vi "Thorlabs-Time Out Check.vi"(8 "error in (no error)":errorcluster, 11 "pDataBuffer in":u16[](array[numeric])) -> (0 "error out":errorcluster, 3 "pDataBuffer out":u16[](array[numeric]))   [LabVIEW 2020]
uses:
  LSM_SDK/ThorConfocal.lvlib
  ECU_SDK/ThorECU.lvlib
panel:
  # "Check that the connection to the scanner is OK"
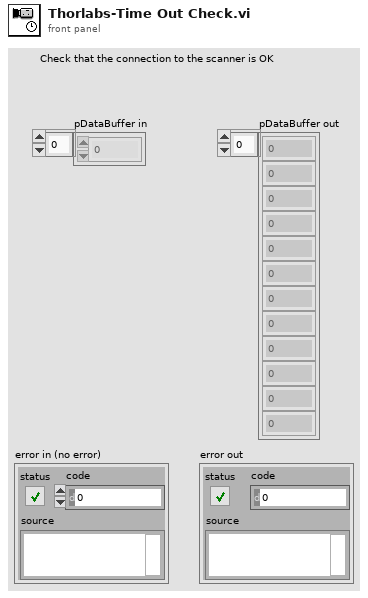
[diagram p1: front panel]
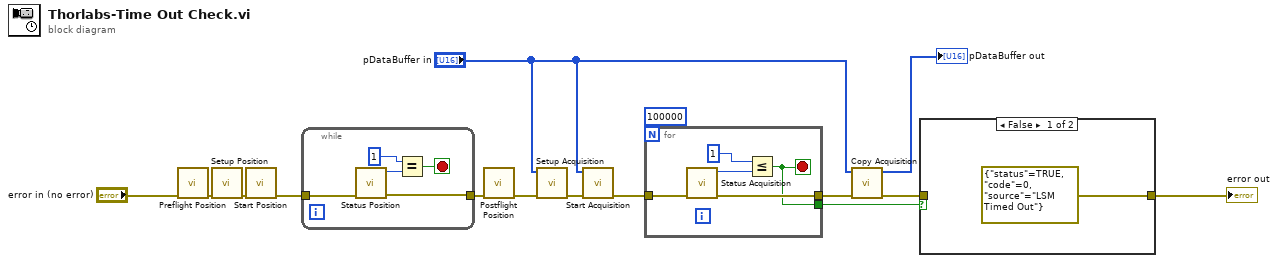
[diagram p0: block diagram]
diagram:
  n1 = call "Preflight Position.vi"("error in (no error)"="error in (no error)") -> ("error out"=w10:errorcluster)  [unwired: 9 in, 1 out]
  n2 = call "Setup Position.vi"("error in (no error)"=w10) -> ("error out"=w11:errorcluster)  [unwired: 9 in, 1 out]
  n3 = call "Start Position.vi"("error in (no error)"=w11) -> ("error out"=w9:errorcluster)  [unwired: 9 in, 1 out]
  n4 = while {
    tunnel: w9 -> [w20]
    tunnel: [w19] -> w8
    stop <- w17 stop-if-true
    n5 = call "Status Position.vi"("error in (no error)"=w20) -> ("error out"=w19:errorcluster, "status out"=w16:i32)  [unwired: 8 in, 1 out]
    n6 = Equal?(x=1, y=w16) -> (x = y?=w17:bool)
  }
  n7 = call "Postflight Position.vi"("error in (no error)"=w8) -> ("error out"=w7:errorcluster)  [unwired: 9 in, 1 out]
  n8 = call "Setup Acquisition.vi"("error in (no error)"=w7, "pDataBuffer"="pDataBuffer in") -> ("error out"=w13:errorcluster)  [unwired: 3 in, 2 out]
  n9 = call "Start Acquisition.vi"("error in (no error)"=w13, "pDataBuffer"="pDataBuffer in") -> ("error out"=w12:errorcluster)  [unwired: 3 in, 2 out]
  n10 = for {
    N: 100000 ("x") -> [_]
    tunnel: [w22] -> w14
    tunnel: w12 -> [w25]
    tunnel: [w21] -> w2
    stop <- w21 stop-if-true
    n11 = call "Status Acquisition.vi"("error in (no error)"=w25) -> ("error out"=w22:errorcluster, "status out"=w23:i32)  [unwired: 4 in, 1 out]
    n12 = Less Or Equal?(x=1, y=w23) -> (x <= y?=w21:bool)
  }
  n13 = call "Copy Acquisition.vi"("error in (no error)"=w14, "pDataBuffer"="pDataBuffer in") -> ("error out"=w4:errorcluster, "pDataBuffer"=→"pDataBuffer out":u16[])  [unwired: 3 in, 1 out]
  n14 = case shown="False" w2 {
    tunnel: [errorcluster {"status"=TRUE, "code"=0, "source"="LSM Timed Out"} ("error constant") w27] -> w5
    tunnel: w4 -> [_ w27]
    frame False {
    }
    frame True {
    }
  }
  "error out" <- w5
